vi "remove-with-tag.vi"(7 "path tag":string="prod", 11 "files found":path[](array[path])) -> (3 "only paths containing tag":path[](array[path]))   [LabVIEW 2014]
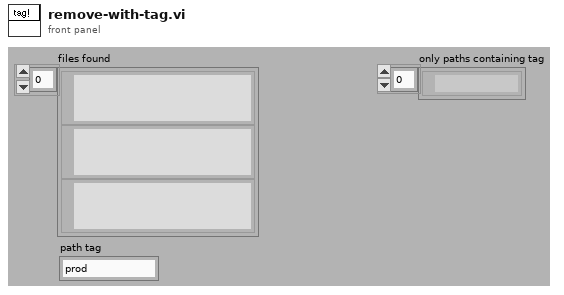
[diagram p1: front panel]
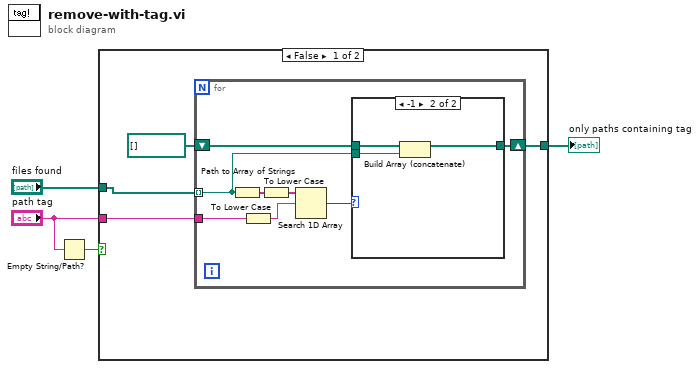
[diagram p0: block diagram]
diagram:
  n1 = Empty String/Path?(string/path="path tag") -> (empty?=w1:bool)
  n2 = case shown="False" w1 {
    tunnel: "files found" -> [w8 w21]
    tunnel: "path tag" -> [w7 _]
    tunnel: [w5 w21] -> w3
    frame False {
      n3 = for {
        tunnel: w8 -> [w13] mode=indexing
        shift-right: [w11] -> w5
        shift-left: path[] [] -> [w12]
        tunnel: w7 -> [w15]
        n4 = Path to Array of Strings(0:w13) -> (2:w16:string[])  [unwired: 1 out]
        n5 = To Lower Case(string=w15) -> (all lower case string=w9:string)
        n6 = To Lower Case(string=w16) -> (all lower case string=w10:string[])
        n7 = Search 1D Array(1D array=w10, element=w9) -> (index of element=w14:i32)  [unwired: 1 out]
        n8 = case shown="-1" w14 {
          tunnel: w13 -> [_ w20]
          tunnel: w12 -> [w17 w19]
          tunnel: [w17 w18] -> w11
          frame 0, Default {
          }
          frame -1 {
            n9 = Build Array (concatenate)(w19, w20) -> (w18:path[])
          }
        }
      }
    }
    frame True {
    }
  }
  "only paths containing tag" <- w3
